vi "JX_SetHome.vi"(8 "error in (no error)":errorcluster, 11 "Jiaxin_Stepper_Controller in":refnum<class "Jiaxin_Stepper_Controller.lvclass">) -> (0 "error out":errorcluster, 3 "Jiaxin_Stepper_Controller out":refnum<class "Jiaxin_Stepper_Controller.lvclass">)   [LabVIEW 2023, in "Jiaxin_Stepper_Controller.lvlib" / "Jiaxin_Stepper_Controller.lvclass"]
uses:
  Jiaxin_Stepper_Controller.lvclass
  Jiaxin_Stepper_Controller.lvclass/Jiaxin_Stepper_Controller.ctl
  Jiaxin_Stepper_Controller.lvlib
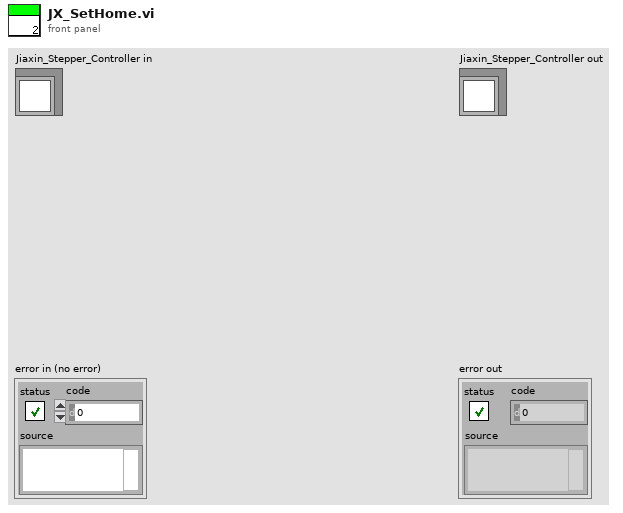
[diagram p1: front panel]
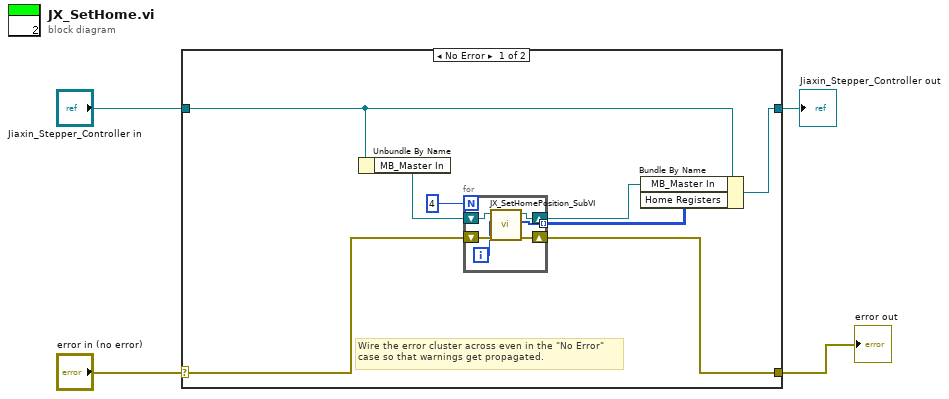
[diagram p0: block diagram]
diagram:
  n1 = case shown="No Error" "error in (no error)" {
    selector: "error in (no error)" -> [w7 w20]
    tunnel: [w6 w20] -> w3
    tunnel: [w8 w19] -> w1
    tunnel: "Jiaxin_Stepper_Controller in" -> [w10 w19]
    frame No Error {
      # "Wire the error cluster across even in the \"No Error\"\ncase so that warnings get propagated."
      n2 = Unbundle By Name(w10) -> ("MB_Master In"=w12:refnum<class "MB_Master.lvclass">)
      n3 = for {
        N: 4 -> [_]
        shift-right: [w15] -> w6
        shift-left: w7 -> [w16]
        tunnel: [w13] -> w5 mode=indexing
        shift-right: [w17] -> w9
        shift-left: w12 -> [w18]
        i -> [w14]
        n4 = call "JX_SetHomePosition_SubVI.vi"("error in (no error)"=w16, "channel"=w14, "Jiaxin_Stepper_Controller.lvlib:MB Serial Master:MB_Master"=w18) -> ("error out"=w15:errorcluster, "Registers"=w13:u16[], "Jiaxin_Stepper_Controller.lvlib:MB Serial Master:MB_Master"=w17:refnum<class "MB_Master.lvclass">)  [unwired: 6 in]
      }
      n5 = Bundle By Name(cluster=w10, "MB_Master In"=w9, "Home Registers"=w5) -> (w8:refnum<class "Jiaxin_Stepper_Controller.lvclass">)
    }
    frame Error {
    }
  }
  "error out" <- w3
  "Jiaxin_Stepper_Controller out" <- w1
